vi "getId.vi"(8 "error in (no error)":errorcluster, 11 "Dot in":refnum<class "Dot.lvclass">) -> (0 "error out":errorcluster, 2 "id":i32, 3 "Dot out":refnum<class "Dot.lvclass">)   [LabVIEW 2018, in "Dot.lvclass"]
uses:
  Dot.lvclass
  Dot.lvclass/Dot.ctl
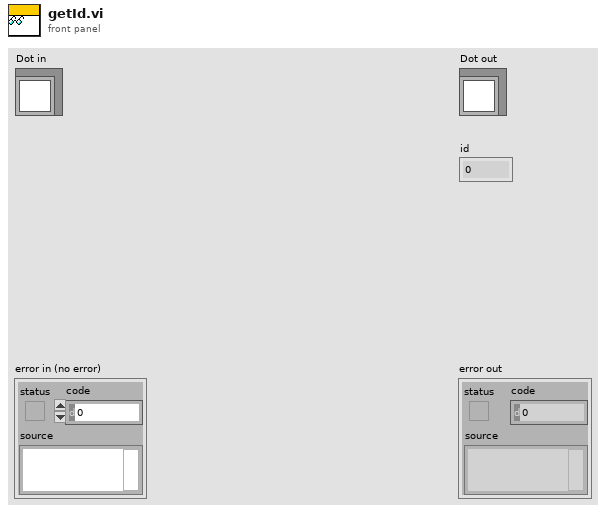
[diagram p1: front panel]
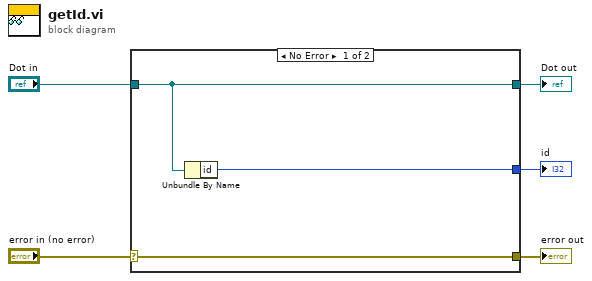
[diagram p0: block diagram]
diagram:
  n1 = case shown="No Error" "error in (no error)" {
    selector: "error in (no error)" -> [w8 w9]
    tunnel: [w8 w9] -> w4
    tunnel: [w7 w10] -> w2
    tunnel: "Dot in" -> [w7 w10]
    tunnel: [w6 _] -> w1
    frame No Error {
      n2 = Unbundle By Name(w7) -> ("id"=w6:i32)
    }
    frame Error {
    }
  }
  "error out" <- w4
  "Dot out" <- w2
  "id" <- w1
